vi "ADC_Dynamic_Input_Parameters.vi"() -> ()   [LabVIEW 2019]
panel:
  in  "Inputs for Dyanmic para":T1={"Fundamental Frequency"=100000.0, "Sampling Frequncy"=3999610.0, "No of Harmonics"=9, "Window"=enum."7 Term B-Harris", "Blackman (fundamental power) bins)"=1.0} {"Blackman (fundamental power) bins)" format="%.2f"; "Sampling Frequncy" format="%^.4e"; "Fundamental Frequency" format="%^.6e"}
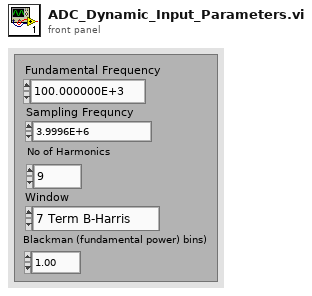
[diagram p1: front panel]
types:
  T1 = cluster{"Fundamental Frequency":dbl, "Sampling Frequncy":dbl, "No of Harmonics":u8, "Window":enum16{"None ", "Hanning", "Hamming", "Blackman-Harris", "Exact Blackman", "Blackman", "Flat Top", "4 Term B-Harris ", "7 Term B-Harris"}, "Blackman (fundamental power) bins)":dbl}
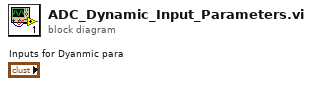
[diagram p0: block diagram]
diagram:
